vi "User Visible Strings.vi"() -> ()   [LabVIEW 2020, in "Text-Based VI Icon.lvlib"]
uses:
  <vilib>/LabVIEW Icon API/Set Text Icon/Text-Based VI Icon.lvlib
panel:
  in  "VI Icon Layer Name":string="VI Icon"
  in  "Class Icon Error":string="Class icon must be a 32-pixel wide rectangle starting at the top row and with at most %d rows. Change class icon before using this function.\n\nClass path: %s"
  in  "Library Icon Error":string="Library icon must be a 32-pixel wide rectangle starting at the top row and with at most %d rows. Change library icon before using this function.\n\nLibrary path: %s"
  in  "Unsaved VI Error":string="Save the VI before using this function."
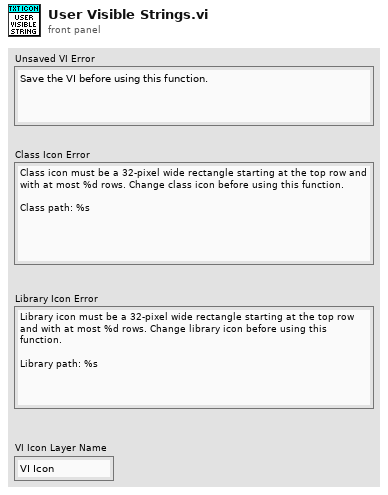
[diagram p1: front panel]
diagram:
